vi "CTRE_Phoenix_MotorControl_ConfigAllSettings_TalonFX.vi"(6 "timeoutMs":i32=50, 7 "Force Write":bool, 8 "error in (no error)":errorcluster, 10 "Talon FX Configurables":T1={"Base Configurables"={"openLoopRamp"=0.0, "closedLoopRamp"=0.0, "peakOutputForward"=1.0, "peakOutputReverse"=-1.0, "nominalOutputForward"=0.0, "nominalOutputReverse"=0.0, "neutralDeadband"=0.04, "voltageCompSaturation"=0.0, "voltageMeasurementFilter"=32, "velocityMeasurementPeriod"=100, "velocityMeasurementWindow"=64, "forwardSoftLimitThreshold"=0, "reverseSoftLimitThreshold"=0, "forwardSoftLimitEnable"=FALSE, "reverseSoftLimitEnable"=FALSE, "slot0"={"P"=0.0, "I"=0.0, "D"=0.0, "F"=0.0, "integralZone"=0.0, "allowableClosedLoopError"=0, "maxIntegralAccumulator"=0.0, "closedLoopPeakOutput"=1.0, "closedLoopPeriod"=1}, "slot1"={"P"=0.0, "I"=0.0, "D"=0.0, "F"=0.0, "integralZone"=0.0, "allowableClosedLoopError"=0, "maxIntegralAccumulator"=0.0, "closedLoopPeakOutput"=1.0, "closedLoopPeriod"=1}, "slot2"={"P"=0.0, "I"=0.0, "D"=0.0, "F"=0.0, "integralZone"=0.0, "allowableClosedLoopError"=0, "maxIntegralAccumulator"=0.0, "closedLoopPeakOutput"=1.0, "closedLoopPeriod"=1}, "slot3"={"P"=0.0, "I"=0.0, "D"=0.0, "F"=0.0, "integralZone"=0.0, "allowableClosedLoopError"=0, "maxIntegralAccumulator"=0.0, "closedLoopPeakOutput"=1.0, "closedLoopPeriod"=1}, "auxPIDPolarity"=FALSE, "remoteFilter0"={"remoteSensorDeviceID"=0, "remoteSensorSource"=enum."Off"}, "remoteFilter1"={"remoteSensorDeviceID"=0, "remoteSensorSource"=enum."Off"}, "motionCruiseVelocity"=0, "motionAcceleration"=0, "motionProfileTrajectoryPeriod"=0, "feedbackNotContinuous"=FALSE, "remoteSensorClosedLoopDisableNeutralOnLOS"=FALSE, "clearPositionOnLimitF"=FALSE, "clearPositionOnLimitR"=FALSE, "clearPositionOnQuadIdx"=FALSE, "limitSwitchDisableNeutralOnLOS"=FALSE, "softLimitDisableNeutralOnLOS"=FALSE, "pulseWidthPeriod_EdgesPerRot"=1, "pulseWidthPeriod_FilterWindowSz"=1, "customParam"={"customParam0"=0, "customParam1"=0}, "trajectoryInterpolationEnable"=TRUE}, "primaryPID"={"selectedFeedbackCoefficient"=1.0, "selectedFeedbackSensor"=1}, "auxiliaryPID"={"selectedFeedbackCoefficient"=1.0, "selectedFeedbackSensor"=1}, "forwardLimitSwitchNormal"=enum."Normally Open", "reverseLimitSwitchNormal"=enum."Normally Open", "forwardLimitSwitchDeviceID"=0, "reverseLimitSwitchDeviceID"=0, "forwardLimitSwitchSource"=enum."Feedback Connector", "reverseLimitSwitchSource"=enum."Feedback Connector", "sum0Term"=1, "sum1Term"=1, "diff0Term"=1, "diff1Term"=1, "Supply Current Limit Configuration"={"Enable?"=FALSE, "Current Limit"=0.0, "Threshold Current"=0.0, "Threshold Time"=0.0}, "Stator Current Limit Configuration"={"Enable?"=FALSE, "Current Limit"=0.0, "Threshold Current"=0.0, "Threshold Time"=0.0}, "Motor Commutation"=enum."Trapezoidal", "Absolute Sensor Range"=enum."Unsigned [0 to 360)", "Integrated Sensor Offset (Degrees)"=0.0, "Sensor Initialization Strategy"=enum."Boot To Zero"} {"diff1Term" items=["Integrated Sensor"=1, "Sensor Sum (S0 + S1)"=9, "Sensor Difference (D0 - D1)"=10, "Remote Source 0"=11, "Remote Source 1"=12, "None"=14, "Software Emulated"=15]; "diff0Term" items=["Integrated Sensor"=1, "Sensor Sum (S0 + S1)"=9, "Sensor Difference (D0 - D1)"=10, "Remote Source 0"=11, "Remote Source 1"=12, "None"=14, "Software Emulated"=15]; "sum1Term" items=["Integrated Sensor"=1, "Sensor Sum (S0 + S1)"=9, "Sensor Difference (D0 - D1)"=10, "Remote Source 0"=11, "Remote Source 1"=12, "None"=14, "Software Emulated"=15]; "sum0Term" items=["Integrated Sensor"=1, "Sensor Sum (S0 + S1)"=9, "Sensor Difference (D0 - D1)"=10, "Remote Source 0"=11, "Remote Source 1"=12, "None"=14, "Software Emulated"=15]; "auxiliaryPID"."selectedFeedbackSensor" items=["Integrated Sensor"=1, "Sensor Sum (S0 + S1)"=9, "Sensor Difference (D0 - D1)"=10, "Remote Source 0"=11, "Remote Source 1"=12, "None"=14, "Software Emulated"=15]; "primaryPID"."selectedFeedbackSensor" items=["Integrated Sensor"=1, "Sensor Sum (S0 + S1)"=9, "Sensor Difference (D0 - D1)"=10, "Remote Source 0"=11, "Remote Source 1"=12, "None"=14, "Software Emulated"=15]; "Base Configurables"."velocityMeasurementPeriod" items=["Period_1ms"=1, "Period_2ms"=2, "Period_5ms"=5, "Period_10ms"=10, "Period_20ms"=20, "Period_25ms"=25, "Period_50ms"=50, "Period_100ms"=100]}, 11 "PhoenixMotorControlDevRef":T16={"DeviceStatus"={"status"=FALSE, "code"=0, "source"=""}, "Type"=enum."PWM", "PWM"={"PWM Channel"=enum."PWM 1", "DeadBand"={"Name"="", "maxPositivePwm"=0, "minPositivePwm"=0, "centerPwm"=0, "maxNegativePwm"=0, "minNegativePwm"=0, "angularRange"=0}}, "CAN"={"Device Number"=0, "SetOutput VI Ref"=variant(enum8{"Percent VBus", "Current", "Speed", "Position", "Voltage"} enum."Percent VBus"), "GetOutput VI Ref"=variant(refnum<k1> refnum), "Enable VI Ref"=variant(dbl 12.0), "Disable VI Ref"=variant(enum8{"Percent VBus", "Speed", "Position", "Slave", "Unchanged / Invalid", "Voltage Compensation", "Current", "Motion Profile"} enum."Percent VBus"), "Data"=variant}, "Invert"=FALSE, "DIO PWM"={"PWM \"Enable\" Channel"=enum."Invalid", "DIOChannel"=enum."Invalid", "PWM Rate"=0.0}}) -> (0 "error out":errorcluster, 3 "PhoenixMotorControlDevRef":T16={"DeviceStatus"={"status"=FALSE, "code"=0, "source"=""}, "Type"=enum."PWM", "PWM"={"PWM Channel"=enum."PWM 1", "DeadBand"={"Name"="", "maxPositivePwm"=0, "minPositivePwm"=0, "centerPwm"=0, "maxNegativePwm"=0, "minNegativePwm"=0, "angularRange"=0}}, "CAN"={"Device Number"=0, "SetOutput VI Ref"=variant(enum8{"Percent VBus", "Current", "Speed", "Position", "Voltage"} enum."Percent VBus"), "GetOutput VI Ref"=variant(refnum<k1> refnum), "Enable VI Ref"=variant(dbl 12.0), "Disable VI Ref"=variant(enum8{"Percent VBus", "Speed", "Position", "Slave", "Unchanged / Invalid", "Voltage Compensation", "Current", "Motion Profile"} enum."Percent VBus"), "Data"=variant}, "Invert"=FALSE, "DIO PWM"={"PWM \"Enable\" Channel"=enum."Invalid", "DIOChannel"=enum."Invalid", "PWM Rate"=0.0}})   [LabVIEW 2019]
doc: "Configures all slot persistant settings\n\n<b>Talon FX Configurables </b> Cluster of all settinsg to be configured"
uses:
  <vilib>/Rock Robotics/WPI/MotorControl/WPI_MotorControlDeviceRef.ctl
  <vilib>/Rock Robotics/WPI/MotorControl/WPI_MotorControlType.ctl
  <vilib>/Rock Robotics/SystemInterfaces/DIO/FPGA_DIOPWMChannel.ctl
  <vilib>/Rock Robotics/WPI/PWM/WPI_PWMDeadband.ctl
  <vilib>/Rock Robotics/SystemInterfaces/DIO/FPGA_DIOChannel.ctl
  <vilib>/Rock Robotics/WPI/ThirdParty/Phoenix-LabVIEW/Motor Controller/Controls/CTRE_Phoenix_MotorControl_TalonFXMotorControllerConfigurables.ctl
  <vilib>/Rock Robotics/WPI/ThirdParty/Phoenix-LabVIEW/Motor Controller/Controls/CTRE_Phoenix_MotorControl_BaseConfigurables.ctl
  <vilib>/Rock Robotics/WPI/ThirdParty/Phoenix-LabVIEW/Motor Controller/Controls/CTRE_Phoenix_MotorControl_VelocityMeasurementPeriod.ctl
  <vilib>/Rock Robotics/WPI/ThirdParty/Phoenix-LabVIEW/Motor Controller/Controls/CTRE_Phoenix_MotorControl_SlotStructure.ctl
  <vilib>/Rock Robotics/WPI/ThirdParty/Phoenix-LabVIEW/Motor Controller/Controls/CTRE_Phoenix_MotorControl_FilterStruct.ctl
  <vilib>/Rock Robotics/WPI/ThirdParty/Phoenix-LabVIEW/Motor Controller/Controls/CTRE_Phoenix_MotorControl_RemoteSourceType.ctl
  <vilib>/Rock Robotics/WPI/ThirdParty/Phoenix-LabVIEW/Controls/CTRE_Phoenix_CustomParamConfiguration.ctl
  <vilib>/Rock Robotics/WPI/ThirdParty/Phoenix-LabVIEW/Motor Controller/Controls/CTRE_Phoenix_MotorControl_FeedbackDevice_TalonFX.ctl
  <vilib>/Rock Robotics/WPI/ThirdParty/Phoenix-LabVIEW/Motor Controller/Controls/CTRE_Phoenix_MotorControl_LimitSwitchNormal.ctl
  <vilib>/Rock Robotics/WPI/ThirdParty/Phoenix-LabVIEW/Motor Controller/Controls/CTRE_Phoenix_MotorControl_LimitSwitchSource_Local.ctl
  <vilib>/Rock Robotics/WPI/ThirdParty/Phoenix-LabVIEW/Motor Controller/Controls/CTRE_Phoenix_MotorControl_SupplyCurrentLimitConfiguration.ctl
  <vilib>/Rock Robotics/WPI/ThirdParty/Phoenix-LabVIEW/Motor Controller/Controls/CTRE_Phoenix_MotorControl_StatorCurrentLimitConfiguration.ctl
  <vilib>/Rock Robotics/WPI/ThirdParty/Phoenix-LabVIEW/Motor Controller/Controls/CTRE_Phoenix_MotorControl_MotorCommutation_TalonFX.ctl
  <vilib>/Rock Robotics/WPI/ThirdParty/Phoenix-LabVIEW/CANCoder/Controls/CTRE_Phoenix_CANcoder_AbsoluteSensorRange.ctl
  <vilib>/Rock Robotics/WPI/ThirdParty/Phoenix-LabVIEW/CANCoder/Controls/CTRE_Phoenix_CANcoder_SensorInitializationStrategy.ctl
panel:
  # "Sum and Diff terms are ways to select more than one sensor as a feedback device. \n Sum 0 is the first feedback device to be used for the Sum term.\n Sum 1 is the feedback device to be added to Sum 0 for the Sum term.\n Diff 0 and Diff 1 work in a similar manner."
  # "These are only applicable\nif using a remote limit switch.\n\nLocal limit switches/no limit\nswitches do not use this."
  # "Current is below Current Limit AND\n\n(Requested output is weaker** than applied motor\noutput OR is in the opposite direction).\n/\nMotor output is set to requested output."
  # "Current is above Threshold Current for Threshold Time\n/\nReduce motor output (towards neutral)."
  # "Current is below Current Limit.\n/\nRamp motor output towards requested output."
  # "Current is above Current Limit.\n/\nReduce motor output (towards neutral)."
  # "*If the configured Peak Threshold is less than the Continuous Threshold, the applied Peak Threshold is set equal to the Configured Continuous Threshold in firmware.\n** Both requested output and applied motor output are in the same direction, and requested output is closer to neutral."
  # "False: Primary Output = PID[0] + PID[1]  ---  Auxiliary Output = PID[0] - PID[1]\nTrue:  Primary Output = PID[0] - PID[1] --- Auxiliary Output = PID[0] + PID[1]"
  # "Enable the motion profile executor to perform linear interpolation between profile points.  Defaults to True."
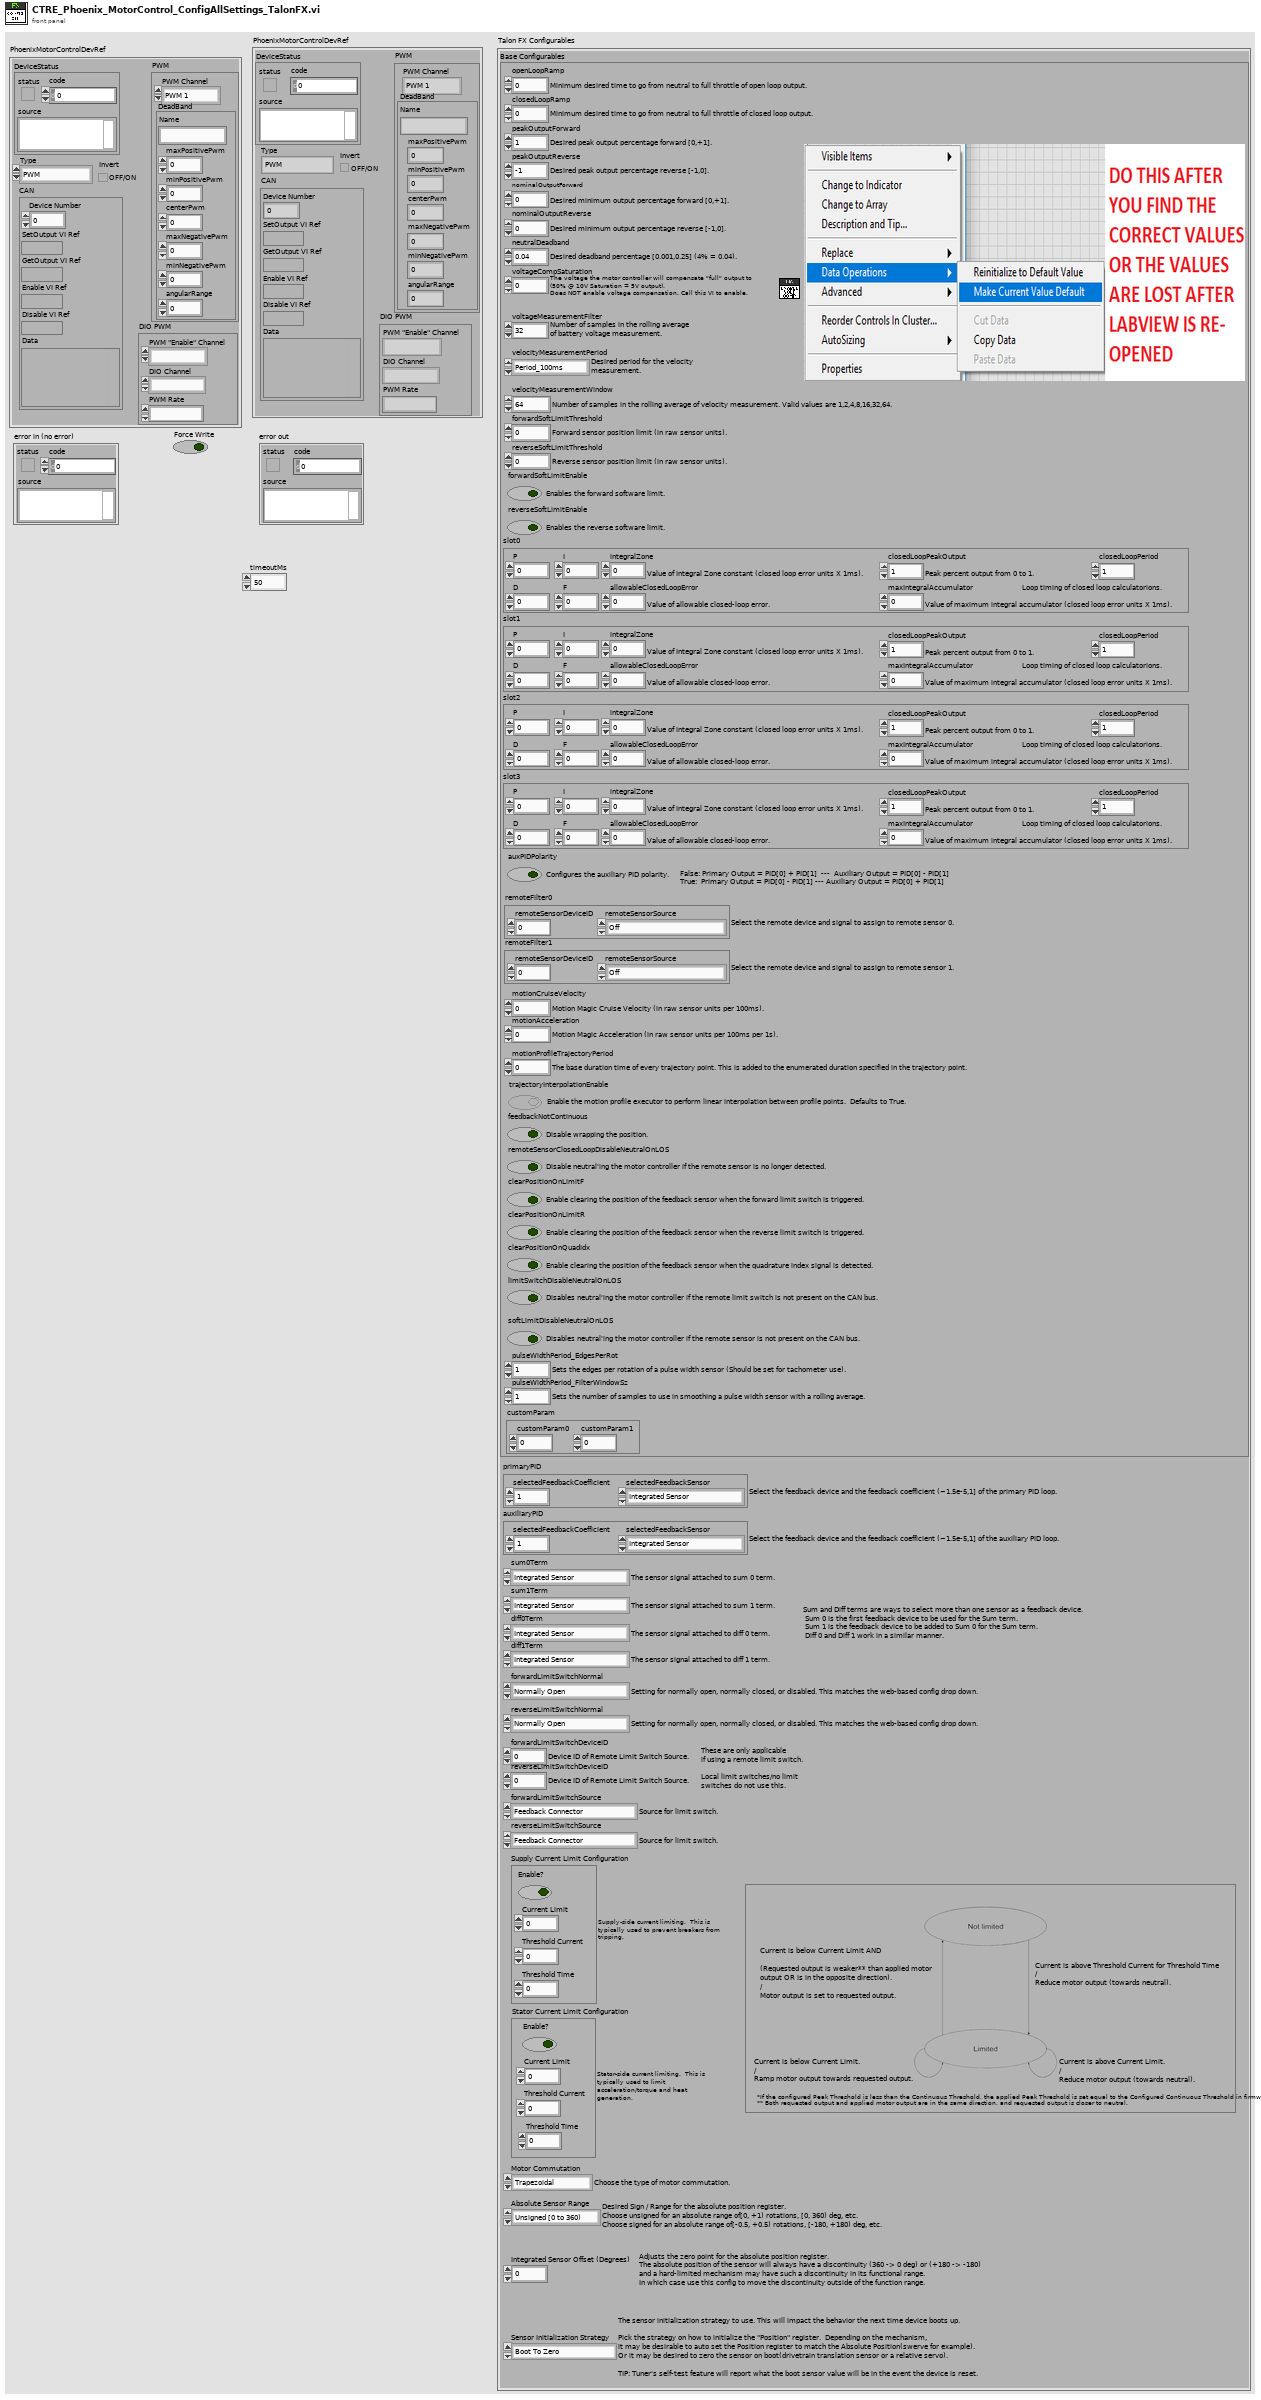
[diagram p1: front panel]
types:
  T1 = typedef "CTRE_Phoenix_MotorControl_TalonFXMotorControllerConfigurables.ctl" = cluster{"Base Configurables":T2, "primaryPID":cluster{"selectedFeedbackCoefficient":dbl, "selectedFeedbackSensor":T8}, "auxiliaryPID":cluster{"selectedFeedbackCoefficient":dbl, "selectedFeedbackSensor":T8}, "forwardLimitSwitchNormal":T9, "reverseLimitSwitchNormal":T9, "forwardLimitSwitchDeviceID":i32, "reverseLimitSwitchDeviceID":i32, "forwardLimitSwitchSource":T10, "reverseLimitSwitchSource":T10, "sum0Term":T8, "sum1Term":T8, "diff0Term":T8, "diff1Term":T8, "Supply Current Limit Configuration":T11, "Stator Current Limit Configuration":T12, "Motor Commutation":T13, "Absolute Sensor Range":T14, "Integrated Sensor Offset (Degrees)":dbl, "Sensor Initialization Strategy":T15}
  T2 = typedef "CTRE_Phoenix_MotorControl_BaseConfigurables.ctl" = cluster{"openLoopRamp":dbl, "closedLoopRamp":dbl, "peakOutputForward":dbl, "peakOutputReverse":dbl, "nominalOutputForward":dbl, "nominalOutputReverse":dbl, "neutralDeadband":dbl, "voltageCompSaturation":dbl, "voltageMeasurementFilter":i32, "velocityMeasurementPeriod":T3, "velocityMeasurementWindow":i32, "forwardSoftLimitThreshold":i32, "reverseSoftLimitThreshold":i32, "forwardSoftLimitEnable":bool, "reverseSoftLimitEnable":bool, "slot0":T4, "slot1":T4, "slot2":T4, "slot3":T4, "auxPIDPolarity":bool, "remoteFilter0":T5, "remoteFilter1":T5, "motionCruiseVelocity":i32, "motionAcceleration":i32, "motionProfileTrajectoryPeriod":i32, "feedbackNotContinuous":bool, "remoteSensorClosedLoopDisableNeutralOnLOS":bool, "clearPositionOnLimitF":bool, "clearPositionOnLimitR":bool, "clearPositionOnQuadIdx":bool, "limitSwitchDisableNeutralOnLOS":bool, "softLimitDisableNeutralOnLOS":bool, "pulseWidthPeriod_EdgesPerRot":i32, "pulseWidthPeriod_FilterWindowSz":i32, "customParam":T7, "trajectoryInterpolationEnable":bool}
  T3 = typedef "CTRE_Phoenix_MotorControl_VelocityMeasurementPeriod.ctl" = u16
  T4 = typedef "CTRE_Phoenix_MotorControl_SlotStructure.ctl" = cluster{"P":dbl, "I":dbl, "D":dbl, "F":dbl, "integralZone":dbl, "allowableClosedLoopError":i32, "maxIntegralAccumulator":dbl, "closedLoopPeakOutput":dbl, "closedLoopPeriod":i32}
  T5 = typedef "CTRE_Phoenix_MotorControl_FilterStruct.ctl" = cluster{"remoteSensorDeviceID":u8, "remoteSensorSource":T6}
  T6 = typedef "CTRE_Phoenix_MotorControl_RemoteSourceType.ctl" = enum16{"Off", "Talon SRX Selected Sensor", "Pigeon IMU Yaw", "Pigeon IMU Pitch", "Pigeon IMU Roll", "CANifier Quadrature", "CANifier PWM Input 0", "CANifier PWM Input 1", "CANifier PWM Input 2", "CANifier PWM Input 3", "Gadgeteer Pigeon Yaw", "Gadgeteer Pigeon Pitch", "Gadgeteer Pigeon Roll"}
  T7 = typedef "CTRE_Phoenix_CustomParamConfiguration.ctl" = cluster{"customParam0":i32, "customParam1":i32}
  T8 = typedef "CTRE_Phoenix_MotorControl_FeedbackDevice_TalonFX.ctl" = i8
  T9 = typedef "CTRE_Phoenix_MotorControl_LimitSwitchNormal.ctl" = enum16{"Normally Open", "Normally Closed", "Disabled"}
  T10 = typedef "CTRE_Phoenix_MotorControl_LimitSwitchSource_Local.ctl" = enum16{"Feedback Connector", "Remote Talon SRX", "Remote CANifier", "Deactivated"}
  T11 = typedef "CTRE_Phoenix_MotorControl_SupplyCurrentLimitConfiguration.ctl" = cluster{"Enable?":bool, "Current Limit":dbl, "Threshold Current":dbl, "Threshold Time":dbl}
  T12 = typedef "CTRE_Phoenix_MotorControl_StatorCurrentLimitConfiguration.ctl" = cluster{"Enable?":bool, "Current Limit":dbl, "Threshold Current":dbl, "Threshold Time":dbl}
  T13 = typedef "CTRE_Phoenix_MotorControl_MotorCommutation_TalonFX.ctl" = enum16{"Trapezoidal"}
  T14 = typedef "CTRE_Phoenix_CANcoder_AbsoluteSensorRange.ctl" = enum16{"Unsigned [0 to 360)", "Signed [-180 to +180)"}
  T15 = typedef "CTRE_Phoenix_CANcoder_SensorInitializationStrategy.ctl" = enum16{"Boot To Zero", "Boot To Absolute Position"}
  T16 = typedef "WPI_MotorControlDeviceRef.ctl" = cluster{"DeviceStatus":errorcluster, "Type":T17, "PWM":cluster{"PWM Channel":T18, "DeadBand":T19}, "CAN":cluster{"Device Number":u8, "SetOutput VI Ref":variant, "GetOutput VI Ref":variant, "Enable VI Ref":variant, "Disable VI Ref":variant, "Data":variant}, "Invert":bool, "DIO PWM":cluster{"PWM \"Enable\" Channel":T18, "DIOChannel":T20, "PWM Rate":dbl}}
  T17 = typedef "WPI_MotorControlType.ctl" = enum16{"PWM", "CAN", "DIO PWM"}
  T18 = typedef "FPGA_DIOPWMChannel.ctl" = enum8{"PWM 0", "PWM 1", "PWM 2", "PWM 3", "PWM 4", "PWM 5", "PWM 6", "PWM 7", "PWM 8", "PWM 9", "PWM MXP 0", "PWM MXP 1", "PWM MXP 2", "PWM MXP 3", "PWM MXP 4", "PWM MXP 5", "PWM MXP 6", "PWM MXP 7", "PWM MXP 8", "PWM MXP 9", "Invalid"}
  T19 = typedef "WPI_PWMDeadband.ctl" = cluster{"Name":string, "maxPositivePwm":i32, "minPositivePwm":i32, "centerPwm":i32, "maxNegativePwm":i32, "minNegativePwm":i32, "angularRange":u16}
  T20 = typedef "FPGA_DIOChannel.ctl" = enum8{"DIO 0", "DIO 1", "DIO 2", "DIO 3", "DIO 4", "DIO 5", "DIO 6", "DIO 7", "DIO 8", "DIO 9", "DIO MXP 0", "DIO MXP 1", "DIO MXP 2", "DIO MXP 3", "DIO MXP 4", "DIO MXP 5", "DIO MXP 6", "DIO MXP 7", "DIO MXP 8", "DIO MXP 9", "DIO MXP 10", "DIO MXP 11", "DIO MXP 12", "DIO MXP 13", "DIO MXP 14", "DIO MXP 15", "SPI Port CS1", "SPI Port CS2", "SPI Port CS3", "SPI Port MISO", "SPI Port MOSI", "Invalid"}
  T21 = cluster{"Base Configurables":cluster{"openLoopRamp":bool, "closedLoopRamp":bool, "peakOutputForward":bool, "peakOutputReverse":bool, "nominalOutputForward":bool, "nominalOutputReverse":bool, "neutralDeadband":bool, "voltageCompSaturation":bool, "voltageMeasurementFilter":bool, "velocityMeasurementPeriod":bool, "velocityMeasurementWindow":bool, "forwardSoftLimitThreshold":bool, "reverseSoftLimitThreshold":bool, "forwardSoftLimitEnable":bool, "reverseSoftLimitEnable":bool, "slot0":cluster{"P":bool, "I":bool, "D":bool, "F":bool, "integralZone":bool, "allowableClosedLoopError":bool, "maxIntegralAccumulator":bool, "closedLoopPeakOutput":bool, "closedLoopPeriod":bool}, "slot1":cluster{"P":bool, "I":bool, "D":bool, "F":bool, "integralZone":bool, "allowableClosedLoopError":bool, "maxIntegralAccumulator":bool, "closedLoopPeakOutput":bool, "closedLoopPeriod":bool}, "slot2":cluster{"P":bool, "I":bool, "D":bool, "F":bool, "integralZone":bool, "allowableClosedLoopError":bool, "maxIntegralAccumulator":bool, "closedLoopPeakOutput":bool, "closedLoopPeriod":bool}, "slot3":cluster{"P":bool, "I":bool, "D":bool, "F":bool, "integralZone":bool, "allowableClosedLoopError":bool, "maxIntegralAccumulator":bool, "closedLoopPeakOutput":bool, "closedLoopPeriod":bool}, "auxPIDPolarity":bool, "remoteFilter0":cluster{"remoteSensorDeviceID":bool, "remoteSensorSource":bool}, "remoteFilter1":cluster{"remoteSensorDeviceID":bool, "remoteSensorSource":bool}, "motionCruiseVelocity":bool, "motionAcceleration":bool, "motionProfileTrajectoryPeriod":bool, "feedbackNotContinuous":bool, "remoteSensorClosedLoopDisableNeutralOnLOS":bool, "clearPositionOnLimitF":bool, "clearPositionOnLimitR":bool, "clearPositionOnQuadIdx":bool, "limitSwitchDisableNeutralOnLOS":bool, "softLimitDisableNeutralOnLOS":bool, "pulseWidthPeriod_EdgesPerRot":bool, "pulseWidthPeriod_FilterWindowSz":bool, "customParam":cluster{"customParam0":bool, "customParam1":bool}, "trajectoryInterpolationEnable":bool}, "primaryPID":cluster{"selectedFeedbackCoefficient":bool, "selectedFeedbackSensor":bool}, "auxiliaryPID":cluster{"selectedFeedbackCoefficient":bool, "selectedFeedbackSensor":bool}, "forwardLimitSwitchNormal":bool, "reverseLimitSwitchNormal":bool, "forwardLimitSwitchDeviceID":bool, "reverseLimitSwitchDeviceID":bool, "forwardLimitSwitchSource":bool, "reverseLimitSwitchSource":bool, "sum0Term":bool, "sum1Term":bool, "diff0Term":bool, "diff1Term":bool, "Supply Current Limit Configuration":cluster{"Enable?":bool, "Current Limit":bool, "Threshold Current":bool, "Threshold Time":bool}, "Stator Current Limit Configuration":cluster{"Enable?":bool, "Current Limit":bool, "Threshold Current":bool, "Threshold Time":bool}, "Motor Commutation":bool, "Absolute Sensor Range":bool, "Integrated Sensor Offset (Degrees)":bool, "Sensor Initialization Strategy":bool}
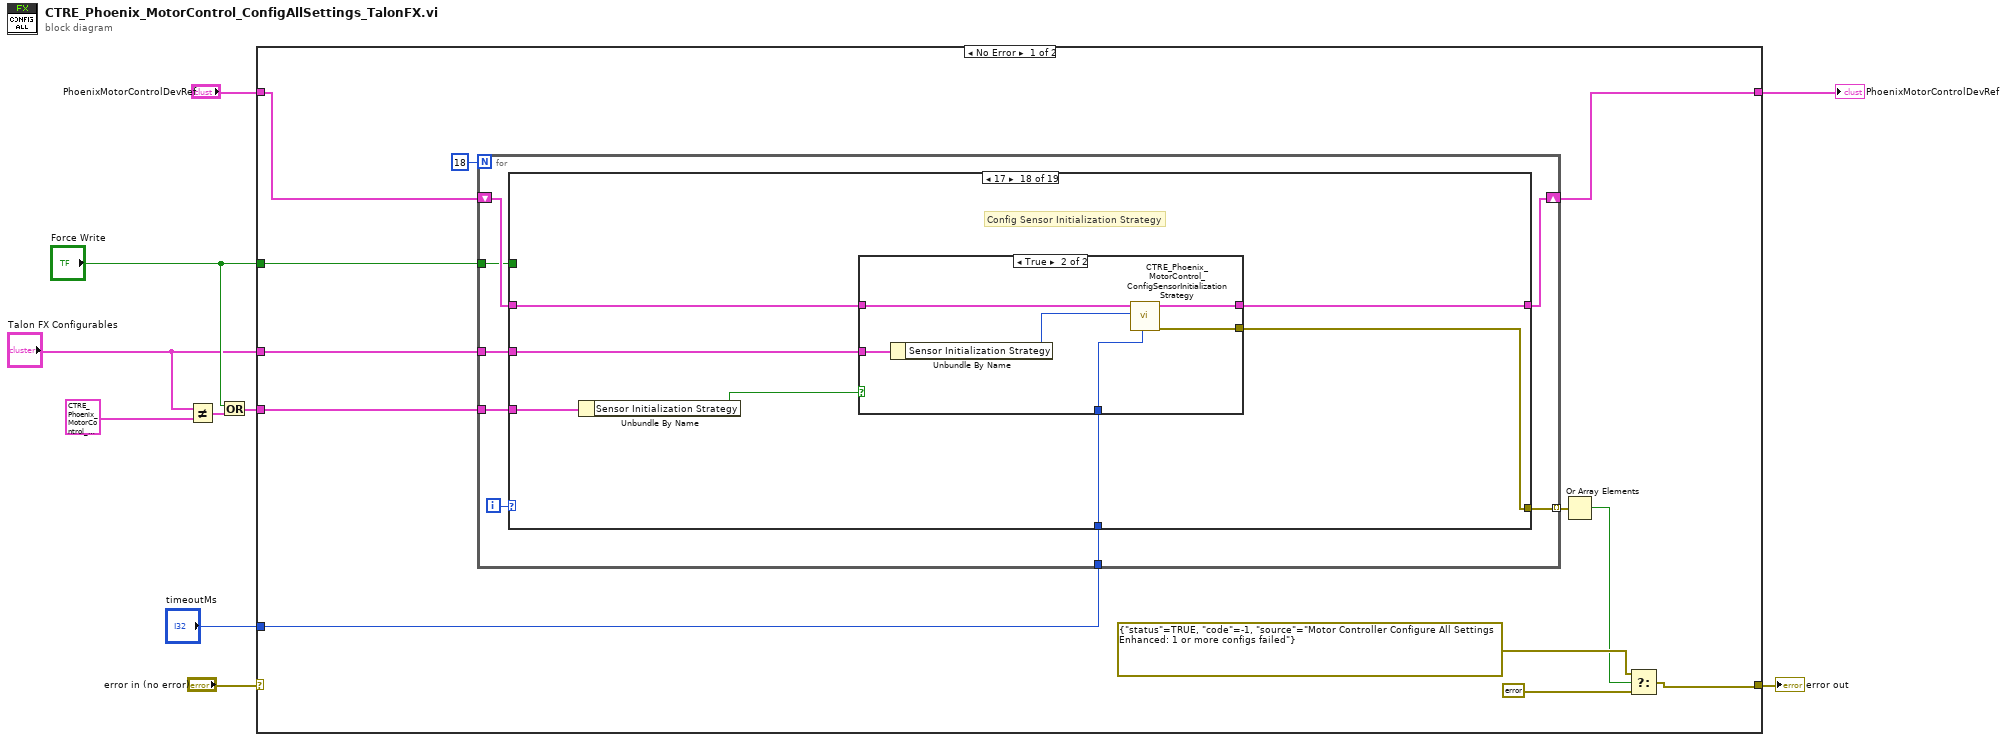
[diagram p0: block diagram]
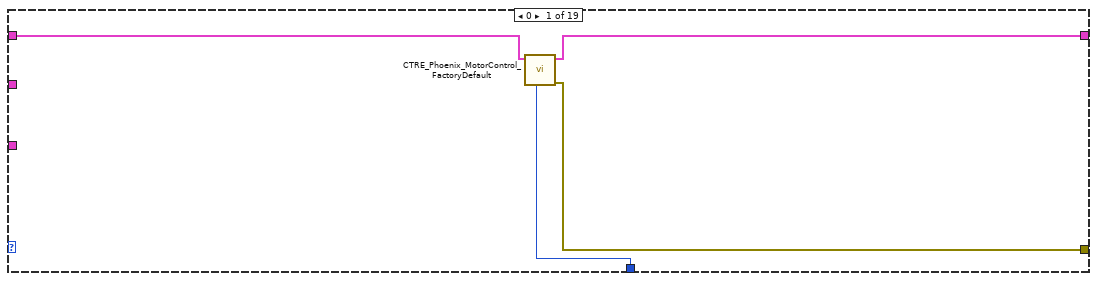
[diagram p2: hidden frame]
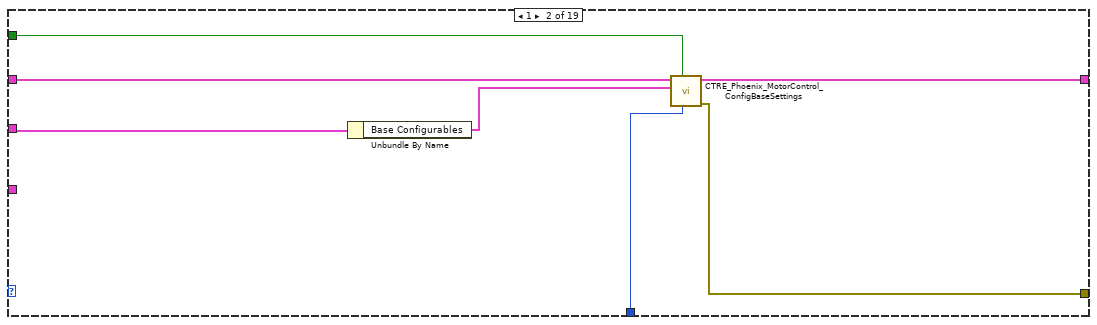
[diagram p3: hidden frame]
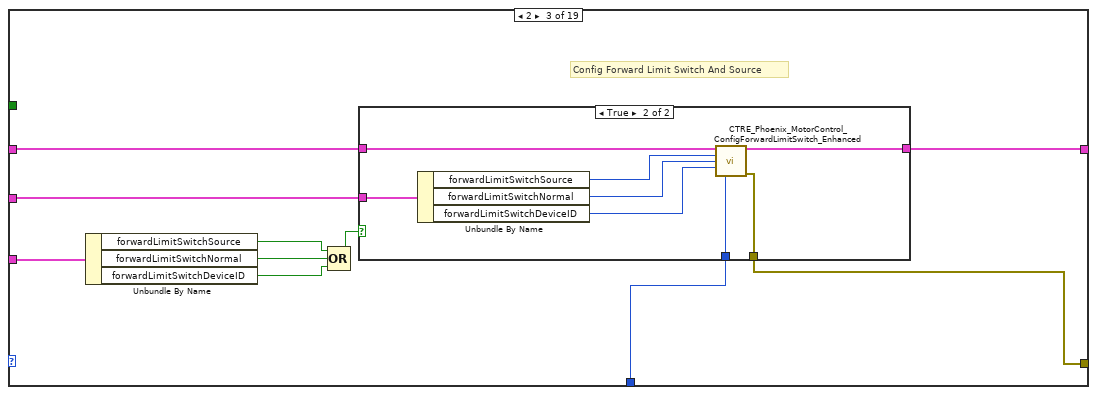
[diagram p4: hidden frame]
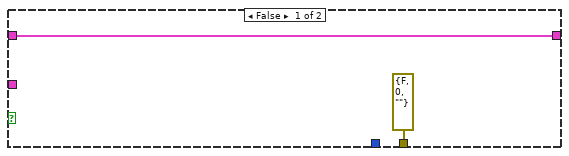
[diagram p5: hidden frame]
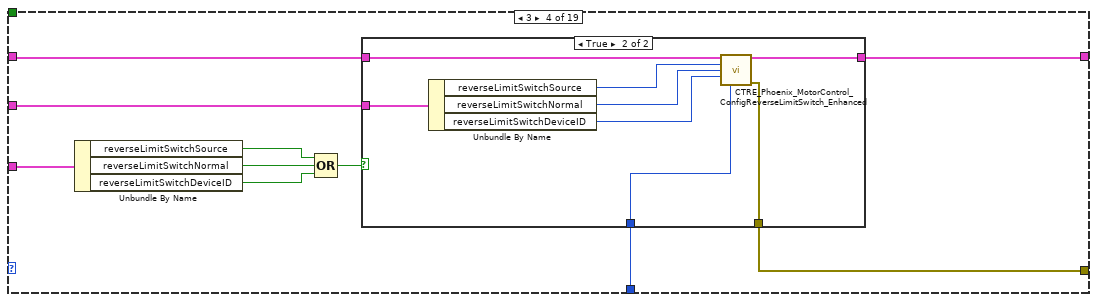
[diagram p6: hidden frame]
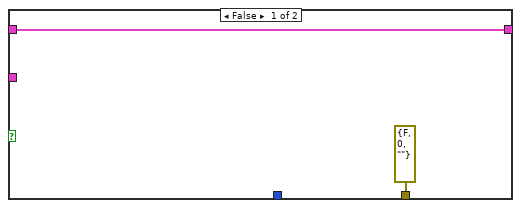
[diagram p7: hidden frame]
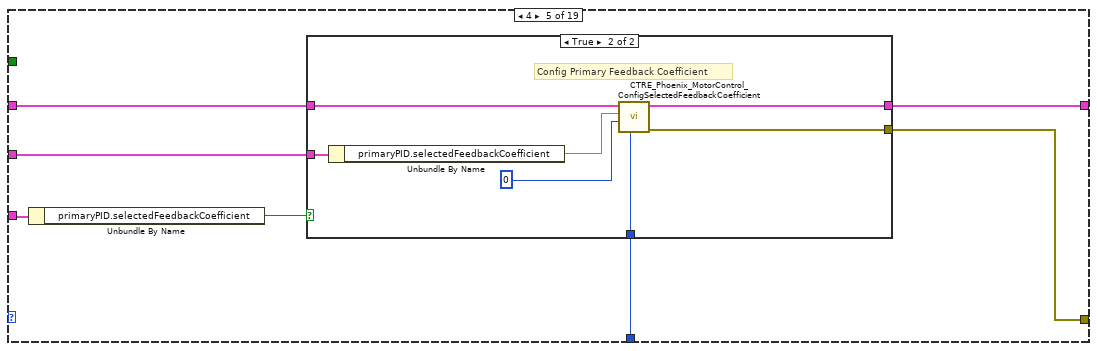
[diagram p8: hidden frame]
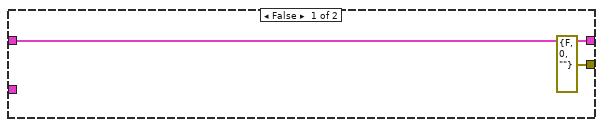
[diagram p9: hidden frame]
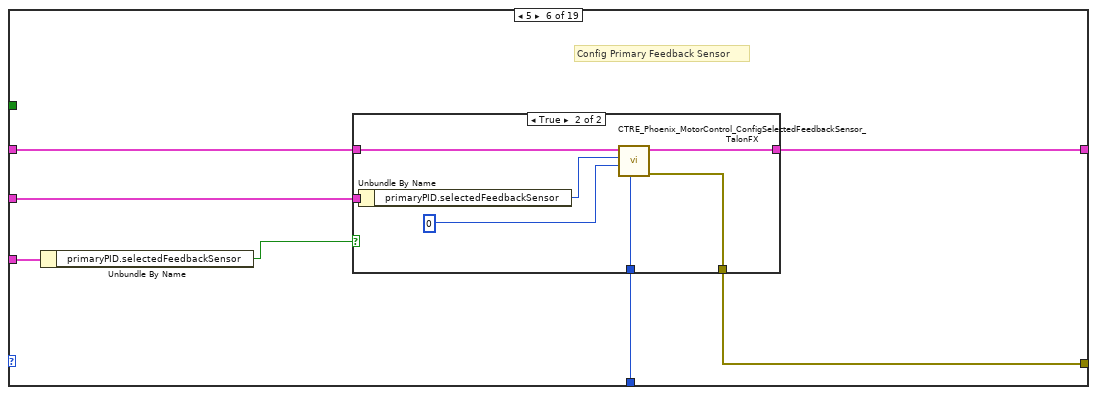
[diagram p10: hidden frame]
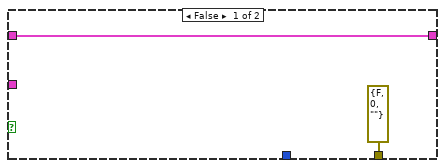
[diagram p11: hidden frame]
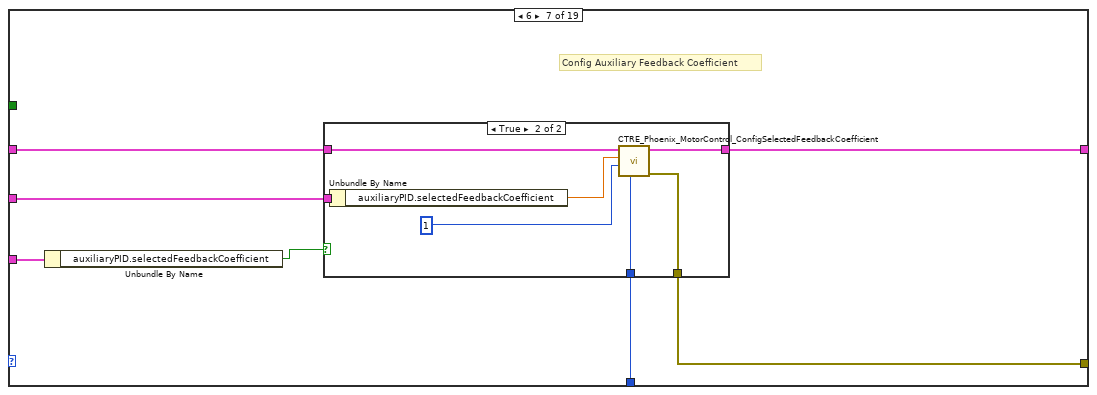
[diagram p12: hidden frame]
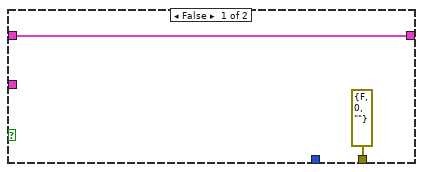
[diagram p13: hidden frame]
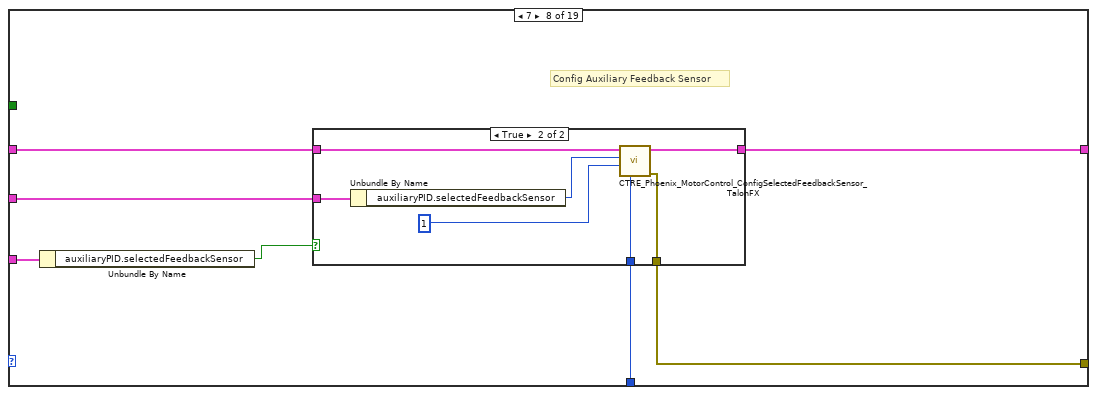
[diagram p14: hidden frame]
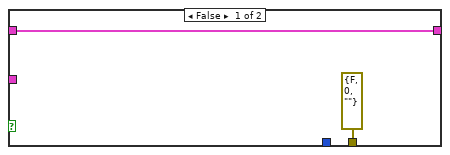
[diagram p15: hidden frame]
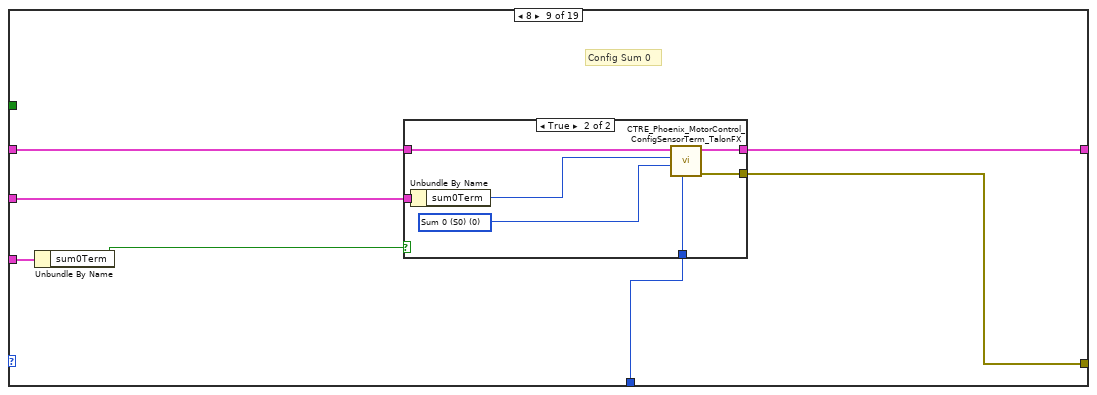
[diagram p16: hidden frame]
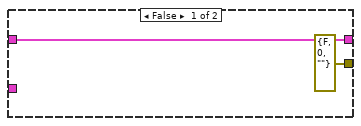
[diagram p17: hidden frame]
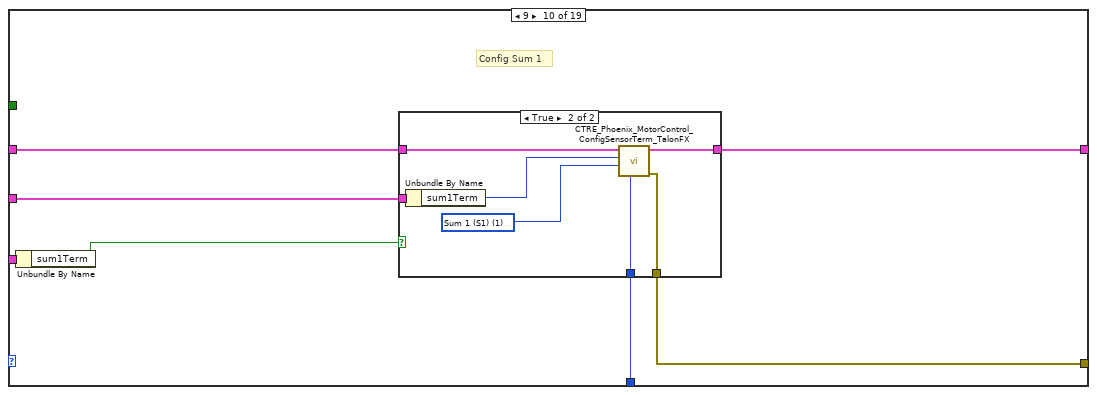
[diagram p18: hidden frame]
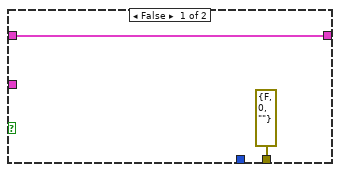
[diagram p19: hidden frame]
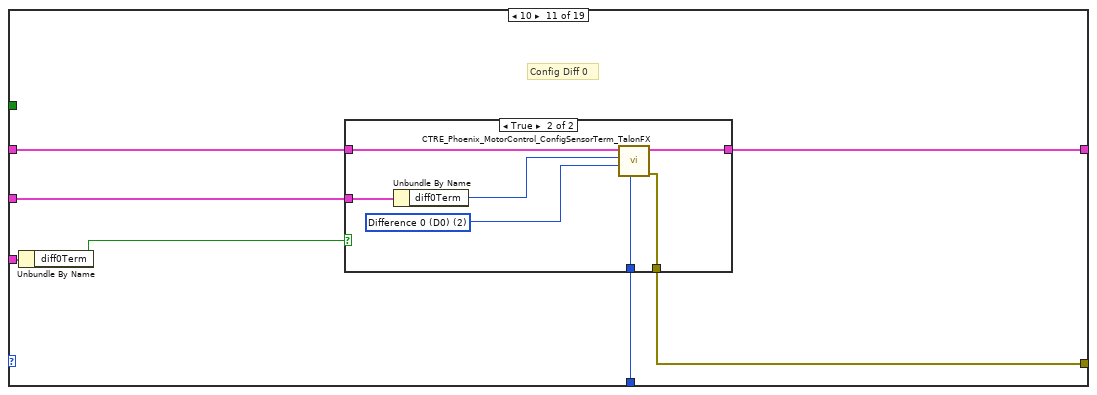
[diagram p20: hidden frame]
diagram:
  n1 = Not Equal?(x="Talon FX Configurables", y=T1 {"Base Configurables"={"openLoopRamp"=0.0, "closedLoopRamp"=0.0, "peakOutputForward"=1.0, "peakOutputReverse"=-1.0, "nominalOutputForward"=0.0, "nominalOutputReverse"=0.0, "neutralDeadband"=0.04, "voltageCompSaturation"=0.0, "voltageMeasurementFilter"=32, "velocityMeasurementPeriod"=100, "velocityMeasurementWindow"=64, "forwardSoftLimitThreshold"=0, "reverseSoftLimitThreshold"=0, "forwardSoftLimitEnable"=FALSE, "reverseSoftLimitEnable"=FALSE, "slot0"={"P"=0.0, "I"=0.0, "D"=0.0, "F"=0.0, "integralZone"=0.0, "allowableClosedLoopError"=0, "maxIntegralAccumulator"=0.0, "closedLoopPeakOutput"=1.0, "closedLoopPeriod"=1}, "slot1"={"P"=0.0, "I"=0.0, "D"=0.0, "F"=0.0, "integralZone"=0.0, "allowableClosedLoopError"=0, "maxIntegralAccumulator"=0.0, "closedLoopPeakOutput"=1.0, "closedLoopPeriod"=1}, "slot2"={"P"=0.0, "I"=0.0, "D"=0.0, "F"=0.0, "integralZone"=0.0, "allowableClosedLoopError"=0, "maxIntegralAccumulator"=0.0, "closedLoopPeakOutput"=1.0, "closedLoopPeriod"=1}, "slot3"={"P"=0.0, "I"=0.0, "D"=0.0, "F"=0.0, "integralZone"=0.0, "allowableClosedLoopError"=0, "maxIntegralAccumulator"=0.0, "closedLoopPeakOutput"=1.0, "closedLoopPeriod"=1}, "auxPIDPolarity"=FALSE, "remoteFilter0"={"remoteSensorDeviceID"=0, "remoteSensorSource"=enum."Off"}, "remoteFilter1"={"remoteSensorDeviceID"=0, "remoteSensorSource"=enum."Off"}, "motionCruiseVelocity"=0, "motionAcceleration"=0, "motionProfileTrajectoryPeriod"=0, "feedbackNotContinuous"=FALSE, "remoteSensorClosedLoopDisableNeutralOnLOS"=FALSE, "clearPositionOnLimitF"=FALSE, "clearPositionOnLimitR"=FALSE, "clearPositionOnQuadIdx"=FALSE, "limitSwitchDisableNeutralOnLOS"=FALSE, "softLimitDisableNeutralOnLOS"=FALSE, "pulseWidthPeriod_EdgesPerRot"=1, "pulseWidthPeriod_FilterWindowSz"=1, "customParam"={"customParam0"=0, "customParam1"=0}, "trajectoryInterpolationEnable"=TRUE}, "primaryPID"={"selectedFeedbackCoefficient"=1.0, "selectedFeedbackSensor"=1}, "auxiliaryPID"={"selectedFeedbackCoefficient"=1.0, "selectedFeedbackSensor"=1}, "forwardLimitSwitchNormal"=enum."Normally Open", "reverseLimitSwitchNormal"=enum."Normally Open", "forwardLimitSwitchDeviceID"=0, "reverseLimitSwitchDeviceID"=0, "forwardLimitSwitchSource"=enum."Feedback Connector", "reverseLimitSwitchSource"=enum."Feedback Connector", "sum0Term"=1, "sum1Term"=1, "diff0Term"=1, "diff1Term"=1, "Supply Current Limit Configuration"={"Enable?"=FALSE, "Current Limit"=0.0, "Threshold Current"=0.0, "Threshold Time"=0.0}, "Stator Current Limit Configuration"={"Enable?"=FALSE, "Current Limit"=0.0, "Threshold Current"=0.0, "Threshold Time"=0.0}, "Motor Commutation"=enum."Trapezoidal", "Absolute Sensor Range"=enum."Unsigned [0 to 360)", "Integrated Sensor Offset (Degrees)"=0.0, "Sensor Initialization Strategy"=enum."Boot To Zero"} ("Talon FX Configurables")) -> (x != y?=w4:T21)
  n2 = Or(x="Force Write", y=w4) -> (x .or. y?=w5:T21)
  n3 = case shown="No Error" "error in (no error)" {
    selector: "error in (no error)" -> [_ w311]
    tunnel: [w22 w311] -> w10
    tunnel: "PhoenixMotorControlDevRef" -> [w18 w310]
    tunnel: [w13 w310] -> w6
    tunnel: "timeoutMs" -> [w17 _]
    tunnel: "Talon FX Configurables" -> [w19 _]
    tunnel: "Force Write" -> [w12 _]
    tunnel: w5 -> [w11 _]
    frame No Error {
      n4 = for {
        N: 18 -> [_]
        tunnel: w19 -> [w30]
        tunnel: w17 -> [w28]
        tunnel: [w26] -> w16 mode=indexing
        shift-right: [w27] -> w13
        shift-left: w18 -> [w29]
        tunnel: w12 -> [w24]
        tunnel: w11 -> [w23]
        i -> [w25]
        n5 = case shown="17" w25 {
          tunnel: w29 -> [w34 w40 w50 w71 w87 w103 w120 w135 w151 w167 w184 w200 w220 w238 w253 w268 w283 w298 w309]
          tunnel: [w33 w41 w47 w67 w86 w102 w119 w136 w150 w165 w183 w197 w219 w237 w252 w267 w282 w297 w309] -> w27
          tunnel: w28 -> [w32 w37 w49 w69 w84 w101 w117 w132 w149 w166 w182 w198 w217 w235 w250 w265 w280 w295 _]
          tunnel: w30 -> [_ w39 w51 w70 w88 w104 w118 w134 w152 w168 w180 w199 w218 w239 w254 w269 w284 w299 _]
          tunnel: [w31 w35 w48 w68 w85 w100 w116 w133 w148 w164 w181 w196 w216 w236 w251 w266 w281 w296 errorcluster {"status"=FALSE, "code"=0, "source"=""} ("error out")] -> w26
          tunnel: w24 -> [_ w36 _ _ _ _ _ _ _ _ _ _ _ _ _ _ _ _ _]
          tunnel: w23 -> [_ _ w46 w66 w83 w99 w115 w131 w147 w163 w179 w195 w210 w234 w249 w264 w279 w294 _]
          frame 0 {
            n6 = call <vilib>:"CTRE_Phoenix_MotorControl_FactoryDefault.vi"("timeoutMs"=w32, "PhoenixMotorControlDevRef"=w34) -> ("error out"=w31:errorcluster, "PhoenixMotorControlDevRef"=w33:T16)  [unwired: 8 in]
          }
          frame 1 {
            n7 = Unbundle By Name(w39) -> ("Base Configurables"=w38:T2)
            n8 = call <vilib>:"CTRE_Phoenix_MotorControl_ConfigBaseSettings.vi"("timeoutMs"=w37, "Force Write"=w36, "Base Configurables"=w38, "PhoenixMotorControlDevRef in"=w40) -> ("error out"=w35:errorcluster, "PhoenixMotorControlDevRef out"=w41:T16)  [unwired: 6 in]
          }
          frame 2 {
            # "Config Forward Limit Switch And Source"
            n9 = Unbundle By Name(w46) -> ("forwardLimitSwitchSource"=w44:bool, "forwardLimitSwitchNormal"=w45:bool, "forwardLimitSwitchDeviceID"=w43:bool)
            n10 = Compound Arithmetic op=OR(w44, w45, w43) -> (w42:bool)
            n11 = case shown="True" w42 {
              tunnel: w51 -> [_ w58]
              tunnel: w50 -> [w53 w57]
              tunnel: w49 -> [_ w56]
              tunnel: [errorcluster {"status"=FALSE, "code"=0, "source"=""} ("error out") w55] -> w48
              tunnel: [w53 w54] -> w47
              frame False {
              }
              frame True {
                n12 = Unbundle By Name(w58) -> ("forwardLimitSwitchSource"=w61:T10, "forwardLimitSwitchNormal"=w60:T9, "forwardLimitSwitchDeviceID"=w59:i32)
                n13 = call <vilib>:"CTRE_Phoenix_MotorControl_ConfigForwardLimitSwitch_Enhanced.vi"("PhoenixMotorControlDevRef"=w57, "Limit Switch Source"=w61, "NormallyOpenOrClosed"=w60, "deviceID"=w59, "timeoutMs"=w56) -> ("PhoenixMotorControlDevRef"=w54:T16, "error out"=w55:errorcluster)  [unwired: 9 in]
              }
            }
          }
          frame 3 {
            n14 = Unbundle By Name(w66) -> ("reverseLimitSwitchSource"=w65:bool, "reverseLimitSwitchNormal"=w64:bool, "reverseLimitSwitchDeviceID"=w63:bool)
            n15 = Compound Arithmetic op=OR(w65, w64, w63) -> (w62:bool)
            n16 = case shown="True" w62 {
              tunnel: w71 -> [w73 w78]
              tunnel: w70 -> [_ w77]
              tunnel: w69 -> [_ w76]
              tunnel: [errorcluster {"status"=FALSE, "code"=0, "source"=""} ("error out") w75] -> w68
              tunnel: [w73 w74] -> w67
              frame False {
              }
              frame True {
                n17 = Unbundle By Name(w77) -> ("reverseLimitSwitchSource"=w81:T10, "reverseLimitSwitchNormal"=w80:T9, "reverseLimitSwitchDeviceID"=w79:i32)
                n18 = call <vilib>:"CTRE_Phoenix_MotorControl_ConfigReverseLimitSwitch_Enhanced.vi"("PhoenixMotorControlDevRef"=w78, "Limit Switch Source"=w81, "NormallyOpenOrClosed"=w80, "deviceID"=w79, "timeoutMs"=w76) -> ("PhoenixMotorControlDevRef"=w74:T16, "error out"=w75:errorcluster)  [unwired: 9 in]
              }
            }
          }
          frame 4 {
            n19 = Unbundle By Name(w83) -> ("primaryPID.selectedFeedbackCoefficient"=w82:bool)
            n20 = case shown="True" w82 {
              tunnel: w88 -> [_ w97]
              tunnel: w87 -> [w90 w96]
              tunnel: [w90 w94] -> w86
              tunnel: [errorcluster {"status"=FALSE, "code"=0, "source"=""} ("error out") w93] -> w85
              tunnel: w84 -> [_ w92]
              frame False {
              }
              frame True {
                # "Config Primary Feedback Coefficient"
                n21 = Unbundle By Name(w97) -> ("primaryPID.selectedFeedbackCoefficient"=w95:dbl)
                n22 = call <vilib>:"CTRE_Phoenix_MotorControl_ConfigSelectedFeedbackCoefficient.vi"("timoutMs"=w92, "pidIdx"=0, "coefficient"=w95, "PhoenixMotorControlDevRef"=w96) -> ("error out"=w93:errorcluster, "PhoenixMotorControlDevRef"=w94:T16)  [unwired: 6 in]
              }
            }
          }
          frame 5 {
            # "Config Primary Feedback Sensor"
            n23 = Unbundle By Name(w99) -> ("primaryPID.selectedFeedbackSensor"=w98:bool)
            n24 = case shown="True" w98 {
              tunnel: w104 -> [_ w113]
              tunnel: w103 -> [w106 w112]
              tunnel: [w106 w111] -> w102
              tunnel: w101 -> [_ w109]
              tunnel: [errorcluster {"status"=FALSE, "code"=0, "source"=""} ("error out") w110] -> w100
              frame False {
              }
              frame True {
                n25 = Unbundle By Name(w113) -> ("primaryPID.selectedFeedbackSensor"=w107:T8)
                n26 = call <vilib>:"CTRE_Phoenix_MotorControl_ConfigSelectedFeedbackSensor_TalonFX.vi"("timeoutMs"=w109, "pidLoopIdx"=0, "Talon FX Feedback Device"=w107, "PhoenixMotorControlDevRef"=w112) -> ("error out"=w110:errorcluster, "PhoenixMotorControlDevRef"=w111:T16)  [unwired: 6 in]
              }
            }
          }
          frame 6 {
            # "Config Auxiliary Feedback Coefficient"
            n27 = Unbundle By Name(w115) -> ("auxiliaryPID.selectedFeedbackCoefficient"=w114:bool)
            n28 = case shown="True" w114 {
              tunnel: w120 -> [w122 w127]
              tunnel: [w122 w126] -> w119
              tunnel: w118 -> [_ w125]
              tunnel: w117 -> [_ w124]
              tunnel: [errorcluster {"status"=FALSE, "code"=0, "source"=""} ("error out") w123] -> w116
              frame False {
              }
              frame True {
                n29 = Unbundle By Name(w125) -> ("auxiliaryPID.selectedFeedbackCoefficient"=w129:dbl)
                n30 = call <vilib>:"CTRE_Phoenix_MotorControl_ConfigSelectedFeedbackCoefficient.vi"("timoutMs"=w124, "pidIdx"=1, "coefficient"=w129, "PhoenixMotorControlDevRef"=w127) -> ("error out"=w123:errorcluster, "PhoenixMotorControlDevRef"=w126:T16)  [unwired: 6 in]
              }
            }
          }
          frame 7 {
            # "Config Auxiliary Feedback Sensor"
            n31 = Unbundle By Name(w131) -> ("auxiliaryPID.selectedFeedbackSensor"=w130:bool)
            n32 = case shown="True" w130 {
              tunnel: [w138 w143] -> w136
              tunnel: w135 -> [w138 w144]
              tunnel: w134 -> [_ w145]
              tunnel: [errorcluster {"status"=FALSE, "code"=0, "source"=""} ("error out") w139] -> w133
              tunnel: w132 -> [_ w140]
              frame False {
              }
              frame True {
                n33 = Unbundle By Name(w145) -> ("auxiliaryPID.selectedFeedbackSensor"=w142:T8)
                n34 = call <vilib>:"CTRE_Phoenix_MotorControl_ConfigSelectedFeedbackSensor_TalonFX.vi"("timeoutMs"=w140, "pidLoopIdx"=1, "Talon FX Feedback Device"=w142, "PhoenixMotorControlDevRef"=w144) -> ("error out"=w139:errorcluster, "PhoenixMotorControlDevRef"=w143:T16)  [unwired: 6 in]
              }
            }
          }
          frame 8 {
            # "Config Sum 0"
            n35 = Unbundle By Name(w147) -> ("sum0Term"=w146:bool)
            n36 = case shown="True" w146 {
              tunnel: w152 -> [_ w161]
              tunnel: w151 -> [w154 w160]
              tunnel: [w154 w156] -> w150
              tunnel: w149 -> [_ w157]
              tunnel: [errorcluster {"status"=FALSE, "code"=0, "source"=""} ("error out") w155] -> w148
              frame False {
              }
              frame True {
                w158 = u16 0 items=["Sum 0 (S0)", "Sum 1 (S1)", "Difference 0 (D0)", "Difference 1 (D1)"] ("Sensor Term")
                n37 = Unbundle By Name(w161) -> ("sum0Term"=w159:T8)
                n38 = call <vilib>:"CTRE_Phoenix_MotorControl_ConfigSensorTerm_TalonFX.vi"("timeoutMs"=w157, "Sensor Term"=w158, "Talon FX Feedback Device"=w159, "PhoenixMotorControlDevRef"=w160) -> ("error out"=w155:errorcluster, "PhoenixMotorControlDevRef"=w156:T16)  [unwired: 6 in]
              }
            }
          }
          frame 9 {
            # "Config Sum 1"
            n39 = Unbundle By Name(w163) -> ("sum1Term"=w162:bool)
            n40 = case shown="True" w162 {
              tunnel: w168 -> [_ w177]
              tunnel: w167 -> [w170 w176]
              tunnel: w166 -> [_ w172]
              tunnel: [w170 w175] -> w165
              tunnel: [errorcluster {"status"=FALSE, "code"=0, "source"=""} ("error out") w171] -> w164
              frame False {
              }
              frame True {
                w173 = u16 1 items=["Sum 0 (S0)", "Sum 1 (S1)", "Difference 0 (D0)", "Difference 1 (D1)"] ("Sensor Term")
                n41 = Unbundle By Name(w177) -> ("sum1Term"=w174:T8)
                n42 = call <vilib>:"CTRE_Phoenix_MotorControl_ConfigSensorTerm_TalonFX.vi"("timeoutMs"=w172, "Sensor Term"=w173, "Talon FX Feedback Device"=w174, "PhoenixMotorControlDevRef"=w176) -> ("error out"=w171:errorcluster, "PhoenixMotorControlDevRef"=w175:T16)  [unwired: 6 in]
              }
            }
          }
          frame 10 {
            # "Config Diff 0"
            n43 = Unbundle By Name(w179) -> ("diff0Term"=w178:bool)
            n44 = case shown="True" w178 {
              tunnel: w184 -> [w186 w192]
              tunnel: [w186 w191] -> w183
              tunnel: w182 -> [_ w188]
              tunnel: [errorcluster {"status"=FALSE, "code"=0, "source"=""} ("error out") w187] -> w181
              tunnel: w180 -> [_ w193]
              frame False {
              }
              frame True {
                w189 = u16 2 items=["Sum 0 (S0)", "Sum 1 (S1)", "Difference 0 (D0)", "Difference 1 (D1)"] ("Sensor Term")
                n45 = Unbundle By Name(w193) -> ("diff0Term"=w190:T8)
                n46 = call <vilib>:"CTRE_Phoenix_MotorControl_ConfigSensorTerm_TalonFX.vi"("timeoutMs"=w188, "Sensor Term"=w189, "Talon FX Feedback Device"=w190, "PhoenixMotorControlDevRef"=w192) -> ("error out"=w187:errorcluster, "PhoenixMotorControlDevRef"=w191:T16)  [unwired: 6 in]
              }
            }
          }
          frame 11 {
            # "Config Diff 1"
            n47 = Unbundle By Name(w195) -> ("diff1Term"=w194:bool)
            n48 = case shown="True" w194 {
              tunnel: w200 -> [w202 w208]
              tunnel: w199 -> [_ w209]
              tunnel: w198 -> [_ w204]
              tunnel: [w202 w207] -> w197
              tunnel: [errorcluster {"status"=FALSE, "code"=0, "source"=""} ("error out") w203] -> w196
              frame False {
              }
              frame True {
                w205 = u16 3 items=["Sum 0 (S0)", "Sum 1 (S1)", "Difference 0 (D0)", "Difference 1 (D1)"] ("Sensor Term")
                n49 = Unbundle By Name(w209) -> ("diff1Term"=w206:T8)
                n50 = call <vilib>:"CTRE_Phoenix_MotorControl_ConfigSensorTerm_TalonFX.vi"("timeoutMs"=w204, "Sensor Term"=w205, "Talon FX Feedback Device"=w206, "PhoenixMotorControlDevRef"=w208) -> ("error out"=w203:errorcluster, "PhoenixMotorControlDevRef"=w207:T16)  [unwired: 6 in]
              }
            }
          }
          frame 12 {
            # "Config Supply Current Limit"
            n51 = Unbundle By Name(w210) -> ("Supply Current Limit Configuration.Enable?"=w215:bool, "Supply Current Limit Configuration.Current Limit"=w214:bool, "Supply Current Limit Configuration.Threshold Current"=w213:bool, "Supply Current Limit Configuration.Threshold Time"=w212:bool)
            n52 = Compound Arithmetic op=OR(w215, w214, w213, w212) -> (w211:bool)
            n53 = case shown="True" w211 {
              tunnel: w220 -> [w222 w227]
              tunnel: [w222 w226] -> w219
              tunnel: w218 -> [_ w228]
              tunnel: w217 -> [_ w224]
              tunnel: [errorcluster {"status"=FALSE, "code"=0, "source"=""} ("error out") w225] -> w216
              frame False {
              }
              frame True {
                n54 = Unbundle By Name(w228) -> ("Supply Current Limit Configuration"=w223:T11)
                n55 = call <vilib>:"CTRE_Phoenix_MotorControl_ConfigSupplyCurrentLimit.vi"("timeoutMs"=w224, "Supply Current Limit Configuration"=w223, "PhoenixMotorControlDevRef"=w227) -> ("error out"=w225:errorcluster, "PhoenixMotorControlDevRef"=w226:T16)  [unwired: 7 in]
              }
            }
          }
          frame 13 {
            # "Config Stator Current Limit"
            n56 = Unbundle By Name(w234) -> ("Stator Current Limit Configuration.Enable?"=w233:bool, "Stator Current Limit Configuration.Current Limit"=w232:bool, "Stator Current Limit Configuration.Threshold Current"=w231:bool, "Stator Current Limit Configuration.Threshold Time"=w230:bool)
            n57 = Compound Arithmetic op=OR(w233, w232, w231, w230) -> (w229:bool)
            n58 = case shown="True" w229 {
              tunnel: w239 -> [_ w247]
              tunnel: w238 -> [w241 w246]
              tunnel: [w241 w245] -> w237
              tunnel: [errorcluster {"status"=FALSE, "code"=0, "source"=""} ("error out") w244] -> w236
              tunnel: w235 -> [_ w243]
              frame False {
              }
              frame True {
                n59 = Unbundle By Name(w247) -> ("Stator Current Limit Configuration"=w242:T12)
                n60 = call <vilib>:"CTRE_Phoenix_MotorControl_ConfigStatorCurrentLimit.vi"("timeoutMs"=w243, "Stator Current Limit Configuration"=w242, "PhoenixMotorControlDevRef"=w246) -> ("error out"=w244:errorcluster, "PhoenixMotorControlDevRef"=w245:T16)  [unwired: 7 in]
              }
            }
          }
          frame 14 {
            # "Config Motor Commutation"
            n61 = Unbundle By Name(w249) -> ("Motor Commutation"=w248:bool)
            n62 = case shown="True" w248 {
              tunnel: w254 -> [_ w262]
              tunnel: w253 -> [w256 w261]
              tunnel: [w256 w260] -> w252
              tunnel: [errorcluster {"status"=FALSE, "code"=0, "source"=""} ("error out") w258] -> w251
              tunnel: w250 -> [_ w259]
              frame False {
              }
              frame True {
                n63 = Unbundle By Name(w262) -> ("Motor Commutation"=w257:T13)
                n64 = call <vilib>:"CTRE_Phoenix_MotorControl_ConfigMotorCommutation.vi"("timeoutMs"=w259, "Motor Commutation"=w257, "PhoenixMotorControlDevRef"=w261) -> ("error out"=w258:errorcluster, "PhoenixMotorControlDevRef"=w260:T16)  [unwired: 7 in]
              }
            }
          }
          frame 15 {
            # "Config Absolute Sensor Range"
            n65 = Unbundle By Name(w264) -> ("Absolute Sensor Range"=w263:bool)
            n66 = case shown="True" w263 {
              tunnel: w269 -> [_ w277]
              tunnel: w268 -> [w271 w276]
              tunnel: [w271 w275] -> w267
              tunnel: [errorcluster {"status"=FALSE, "code"=0, "source"=""} ("error out") w274] -> w266
              tunnel: w265 -> [_ w273]
              frame False {
              }
              frame True {
                n67 = Unbundle By Name(w277) -> ("Absolute Sensor Range"=w272:T14)
                n68 = call <vilib>:"CTRE_Phoenix_MotorControl_ConfigAbsoluteSensorRange.vi"("timeoutMs"=w273, "Absolute Sensor Range"=w272, "PhoenixMotorControlDevRef"=w276) -> ("error out"=w274:errorcluster, "PhoenixMotorControlDevRef"=w275:T16)  [unwired: 7 in]
              }
            }
          }
          frame 16 {
            # "Config Ingetrated Sensor Offset"
            n69 = Unbundle By Name(w279) -> ("Integrated Sensor Offset (Degrees)"=w278:bool)
            n70 = case shown="True" w278 {
              tunnel: w284 -> [_ w292]
              tunnel: w283 -> [w286 w291]
              tunnel: [w286 w290] -> w282
              tunnel: [errorcluster {"status"=FALSE, "code"=0, "source"=""} ("error out") w287] -> w281
              tunnel: w280 -> [_ w288]
              frame False {
              }
              frame True {
                n71 = Unbundle By Name(w292) -> ("Integrated Sensor Offset (Degrees)"=w289:dbl)
                n72 = call <vilib>:"CTRE_Phoenix_MotorControl_ConfigIntegratedSensorOffset.vi"("timeoutMs"=w288, "Offset (Degrees)"=w289, "PhoenixMotorControlDevRef"=w291) -> ("error out"=w287:errorcluster, "PhoenixMotorControlDevRef"=w290:T16)  [unwired: 7 in]
              }
            }
          }
          frame 17 {
            # "Config Sensor Initialization Strategy"
            n73 = Unbundle By Name(w294) -> ("Sensor Initialization Strategy"=w293:bool)
            n74 = case shown="True" w293 {
              tunnel: w299 -> [_ w307]
              tunnel: w298 -> [w301 w306]
              tunnel: [w301 w305] -> w297
              tunnel: [errorcluster {"status"=FALSE, "code"=0, "source"=""} ("error out") w302] -> w296
              tunnel: w295 -> [_ w303]
              frame False {
              }
              frame True {
                n75 = Unbundle By Name(w307) -> ("Sensor Initialization Strategy"=w304:T15)
                n76 = call <vilib>:"CTRE_Phoenix_MotorControl_ConfigSensorInitializationStrategy.vi"("timeoutMs"=w303, "Sensor Initialization Strategy"=w304, "PhoenixMotorControlDevRef"=w306) -> ("error out"=w302:errorcluster, "PhoenixMotorControlDevRef"=w305:T16)  [unwired: 7 in]
              }
            }
          }
          frame Default {
          }
        }
      }
      n77 = Or Array Elements(Boolean array=w16) -> (logical OR=w15:bool)
      n78 = Select(t=errorcluster {"status"=TRUE, "code"=-1, "source"="Motor Controller Configure All Settings Enhanced: 1 or more configs failed"} ("error out 2"), s=w15, f=errorcluster {"status"=FALSE, "code"=0, "source"=""} ("error out 2")) -> (s? t:f=w22:errorcluster)
    }
    frame Error {
    }
  }
  "PhoenixMotorControlDevRef" <- w6
  "error out" <- w10
